vi "LINC Process Text.vi"(1 "line in":string) -> (0 "line out":string)   [LabVIEW 2018, in "STEPkgDriver_LINC.lvlib"]
uses:
  STEPkgDriver_LINC.lvlib
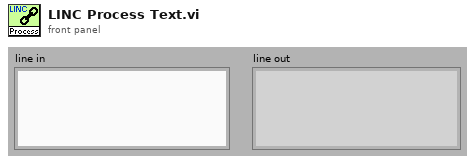
[diagram p1: front panel]
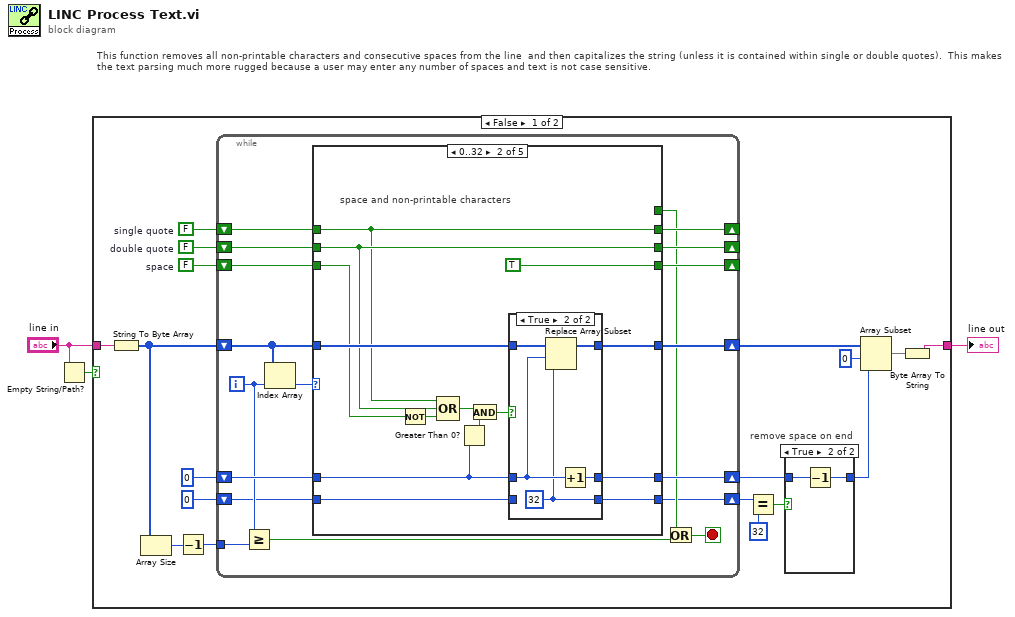
[diagram p0: block diagram]
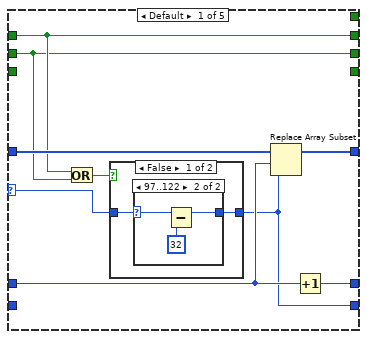
[diagram p2: hidden frame]
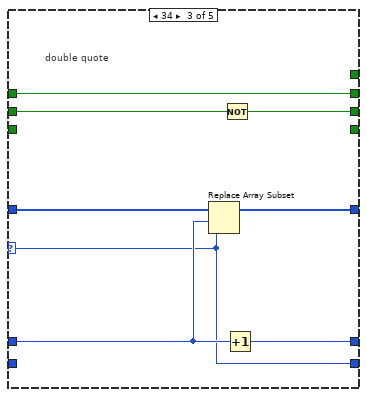
[diagram p6: hidden frame]
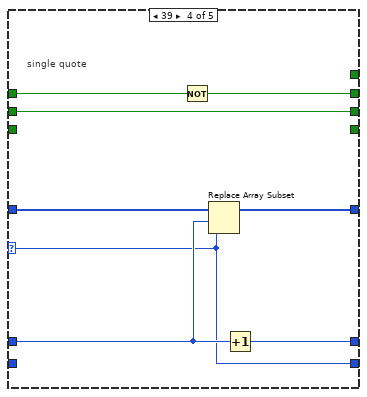
[diagram p7: hidden frame]
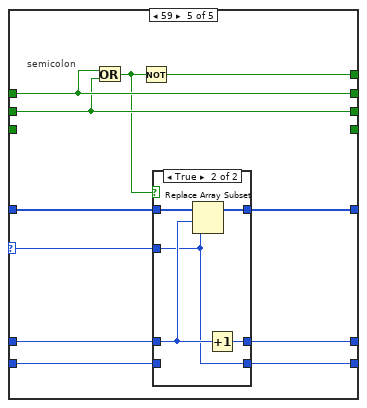
[diagram p8: hidden frame]
diagram:
  # "This function removes all non-printable characters and consecutive spaces from the line  and then capitalizes the string (unless it is contained within single or double quotes).  This makes the text parsing much more rugged because a user may enter any number of spaces and text is not case sensitive."
  n1 = Empty String/Path?(string/path="line in") -> (empty?=w2:bool)
  n2 = case shown="False" w2 {
    tunnel: "line in" -> [w16 w116]
    tunnel: [w14 w116] -> w1
    frame False {
      w13 = FALSE  # single quote
      w15 = FALSE  # space
      w17 = FALSE  # double quote
      # "remove space on end"
      n3 = String To Byte Array(string=w16) -> (unsigned byte array=w18:u8[])
      n4 = Array Size(array=w18) -> (size(s)=w8:i32)
      n5 = Decrement(x=w8) -> (x-1=w7:i32)
      n6 = while {
        shift-right: [w36] -> w19
        shift-left: w18 -> [w39]
        shift-right: [w37] -> w10
        shift-left: 0 -> [w38]
        shift-right: [w34] -> _
        shift-left: w17 -> [w35]
        shift-right: [w32] -> _
        shift-left: w15 -> [w33]
        shift-right: [w31] -> _
        shift-left: w13 -> [w30]
        tunnel: w7 -> [w28]
        shift-right: [w22] -> w4
        shift-left: u8 0 ("new element/subarray") -> [w23]
        i -> [w29]
        stop <- w24 stop-if-true
        n7 = Greater Or Equal?(x=w29, y=w28) -> (x >= y?=w27:bool)
        n8 = Index Array(array=w39, index=w29) -> (element=w26:u8)
        n9 = case shown="0..32" w26 {
          selector: w26 -> [w41 _ w78 w86 w101]
          tunnel: w39 -> [w48 w69 w83 w93 w104]
          tunnel: w38 -> [w46 w63 w81 w91 w102]
          tunnel: [w45 w67 w80 w90 w100] -> w37
          tunnel: [w47 w68 w82 w92 w103] -> w36
          tunnel: w35 -> [w43 w64 w85 w87 w98]
          tunnel: [w43 w64 w84 w87 w98] -> w34
          tunnel: w33 -> [_ w65 _ _ _]
          tunnel: [_ TRUE _ _ _] -> w32
          tunnel: w30 -> [w44 w62 w79 w88 w99]
          tunnel: [w44 w62 w79 w89 w99] -> w31
          tunnel: [_ _ _ _ w96] -> w25
          tunnel: w23 -> [_ w56 _ _ w95]
          tunnel: [w40 w57 w78 w86 w94] -> w22
          frame Default {
            n10 = Or(x=w44, y=w43) -> (x .or. y?=w42:bool)
            n11 = case shown="False" w42 {
              tunnel: w41 -> [w50 w55]
              tunnel: [w49 w55] -> w40
              frame False {
                n12 = case shown="97..122" w50 {
                  selector: w50 -> [w51 w54]
                  tunnel: [w51 w52] -> w49
                  frame Default {
                  }
                  frame 97..122 {
                    n13 = Subtract(x=w54, y=u8 32) -> (x-y=w52:u8)
                  }
                }
              }
              frame True {
              }
            }
            n14 = Replace Array Subset(array=w48, new element=w40, index=w46) -> (w47:u8[])
            n15 = Increment(x=w46) -> (x+1=w45:i32)
          }
          frame 0..32 {
            # "space and non-printable characters"
            n16 = Not(x=w65) -> (.not. x?=w61:bool)
            n17 = Compound Arithmetic op=OR(w62, w64, w61) -> (w60:bool)
            n18 = Greater Than 0?(x=w63) -> (x > 0?=w59:bool)
            n19 = And(x=w60, y=w59) -> (x .and. y?=w58:bool)
            n20 = case shown="True" w58 {
              tunnel: w69 -> [w72 w77]
              tunnel: [w72 w76] -> w68
              tunnel: w63 -> [w71 w75]
              tunnel: [w71 w74] -> w67
              tunnel: [w70 w73] -> w57
              tunnel: w56 -> [w70 _]
              frame False {
              }
              frame True {
                w73 = u8 32 ("new element/subarray")
                n21 = Replace Array Subset(array=w77, new element=w73, index=w75) -> (w76:u8[])
                n22 = Increment(x=w75) -> (x+1=w74:i32)
              }
            }
          }
          frame 34 {
            # "double quote"
            n23 = Replace Array Subset(array=w83, new element=w78, index=w81) -> (w82:u8[])
            n24 = Not(x=w85) -> (.not. x?=w84:bool)
            n25 = Increment(x=w81) -> (x+1=w80:i32)
          }
          frame 39 {
            # "single quote"
            n26 = Not(x=w88) -> (.not. x?=w89:bool)
            n27 = Replace Array Subset(array=w93, new element=w86, index=w91) -> (w92:u8[])
            n28 = Increment(x=w91) -> (x+1=w90:i32)
          }
          frame 59 {
            # "semicolon"
            n29 = Or(x=w99, y=w98) -> (x .or. y?=w97:bool)
            n30 = Not(x=w97) -> (.not. x?=w96:bool)
            n31 = case shown="True" w97 {
              tunnel: w104 -> [w107 w112]
              tunnel: [w107 w111] -> w103
              tunnel: w102 -> [w106 w110]
              tunnel: w101 -> [_ w108]
              tunnel: [w106 w109] -> w100
              tunnel: w95 -> [w105 _]
              tunnel: [w105 w108] -> w94
              frame False {
              }
              frame True {
                n32 = Replace Array Subset(array=w112, new element=w108, index=w110) -> (w111:u8[])
                n33 = Increment(x=w110) -> (x+1=w109:i32)
              }
            }
          }
        }
        n34 = Or(x=w25, y=w27) -> (x .or. y?=w24:bool)
      }
      n35 = Equal?(x=w4, y=u8 32) -> (x = y?=w11:bool)
      n36 = case shown="True" w11 {
        tunnel: w10 -> [w113 w115]
        tunnel: [w113 w114] -> w9
        frame False {
        }
        frame True {
          n37 = Decrement(x=w115) -> (x-1=w114:i32)
        }
      }
      n38 = Array Subset(array=w19, index=0, length=w9) -> (w21:u8[])
      n39 = Byte Array To String(unsigned byte array=w21) -> (string=w14:string)
    }
    frame True {
    }
  }
  "line out" <- w1
